vi "operation.vi"() -> ()   [LabVIEW 2024]
panel:
  out "Vertical Progress Bar":u8(slide) scale=0.0..100.0
  out "x*y":dbl
  in  "y":dbl
  in  "x":dbl
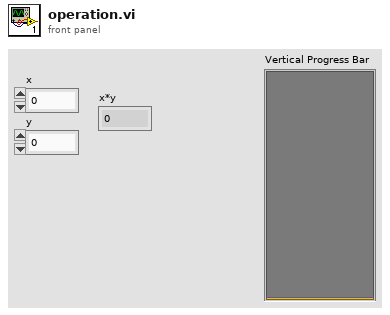
[diagram p1: front panel]
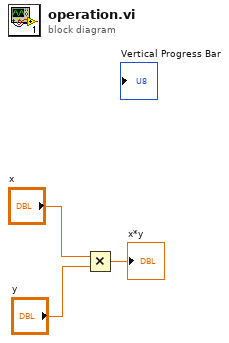
[diagram p0: block diagram]
diagram:
  n1 = Multiply(x="x", y="y") -> (x*y=→"x*y":dbl)
